vi "Main.vi"(11 "Module Admin":refnum<class "Delacor_lib_QMH_Module Admin.lvclass">) -> ()   [LabVIEW 2025, in "Central Monitor.lvlib"]
doc: "This template is based off of the Queued Message Handler design pattern and the Queued Message Handler project template that ships with LabVIEW.\n\nThe main difference is that the queue is private to this module and communication between modules is performed via Broadcast and Request events.\n\nRequest events are wrapped in public API methods and are handled in the Event Handling Loop (EHL) of this VI. Any module can register for Broadcast events sent by this module. The EHL generates messages based on user interface actions.\n\nThe Message Handling Loop (MHL) processes messages generated by the EHL, or by other messages. The messages are string values, so new messages can be added easily to the Message Cases case structure in the MHL. Each message cluster can also provide an optional value for Message Data, which is a variant that can be converted to whatever message-specific data is required.\n_____\nBased on DQMH Dev Tools: Project Template 7.1.2.1547."
uses:
  Central Monitor.lvlib
  <vilib>/Delacor/Delacor QMH/Libraries/Module Admin_class/Delacor_lib_QMH_Module Admin.lvclass
  Module Data--cluster.ctl
  <vilib>/Delacor/Delacor QMH/Libraries/Message Queue_class/Delacor_lib_QMH_Message Queue.lvclass/Delacor_lib_QMH_Message Queue.ctl
  Stop Argument--cluster.ctl
  <vilib>/Delacor/Delacor QMH/Libraries/Module Admin_class/Delacor_lib_QMH_Module Admin.lvclass/Delacor_lib_QMH_Module Admin.ctl
  <vilib>/Utility/miscctls.llb/LVPointTypeDef.ctl
  <vilib>/Delacor/Delacor QMH/Libraries/Message Queue_class/Delacor_lib_QMH_Enqueue Message (Single).vi
  <vilib>/Delacor/Delacor QMH/Libraries/Module Admin_class/Delacor_lib_QMH_Get External Launch.vi
  <vilib>/Delacor/Delacor QMH/Libraries/Message Queue_class/Delacor_lib_QMH_Message Queue.lvclass
panel:
  in  "Multicolumn Listbox":i32(listbox)
  in  "Button":bool
  out "Monitor Status":bool
  out "Headline":string
  out "error out":errorcluster
  out "Status":string
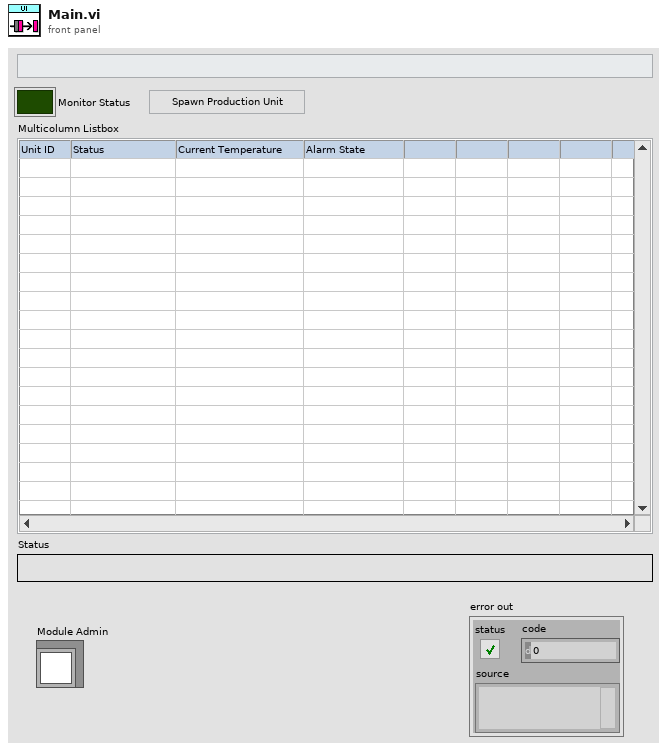
[diagram p1: front panel]
types:
  T1 = typedef "Central Monitor.lvlib/Request Events--cluster.ctl" = cluster{"Stop Module":refnum<user-event>, "Show Panel":refnum<user-event>, "Hide Panel":refnum<user-event>, "Get Module Execution Status":refnum<user-event>, "Show Diagram":refnum<user-event>}
  T2 = typedef "Central Monitor.lvlib/Module Data--cluster.ctl" = cluster{"Status":string}
  T3 = enum32{"invalid lock state", "Not Locked", "Locked (No Password)", "Password-protected"}
  T4 = typedef "Central Monitor.lvlib/Stop Argument--cluster.ctl" = cluster{"Origin":string, "Exit via Stop Module Req?":bool, "Wait for Module to stop?":bool}
  T5 = typedef "LVPointTypeDef.ctl" = cluster{"Horizontal":i16, "Vertical":i16}
  T6 = enum32{"Invalid", "Standard", "Closed", "Hidden", "Minimized", "Maximized"}
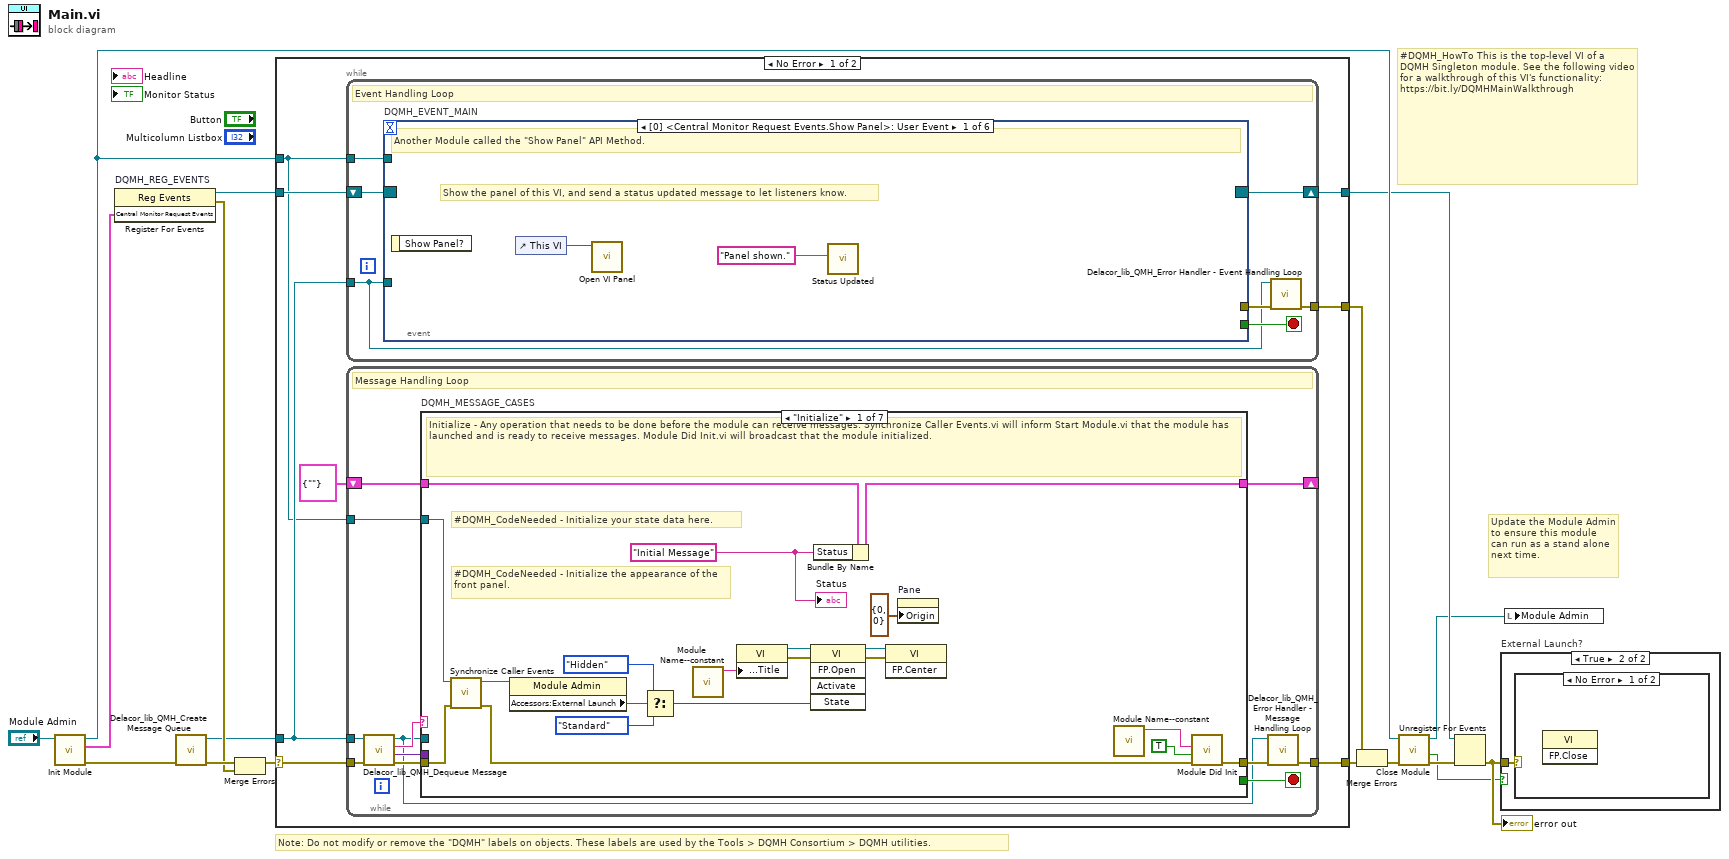
[diagram p0: block diagram]
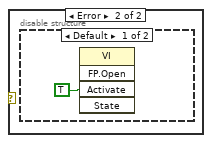
[diagram p3: hidden frame]
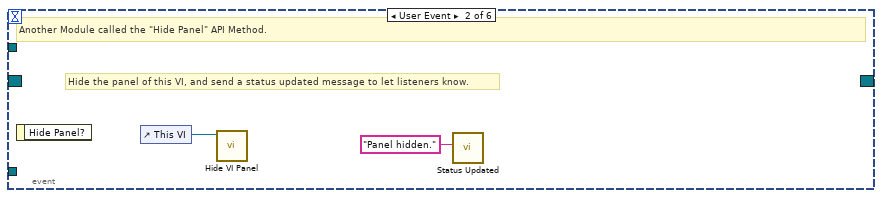
[diagram p5: hidden frame]
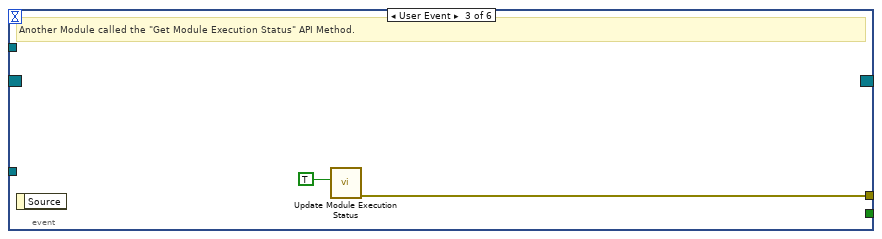
[diagram p6: hidden frame]
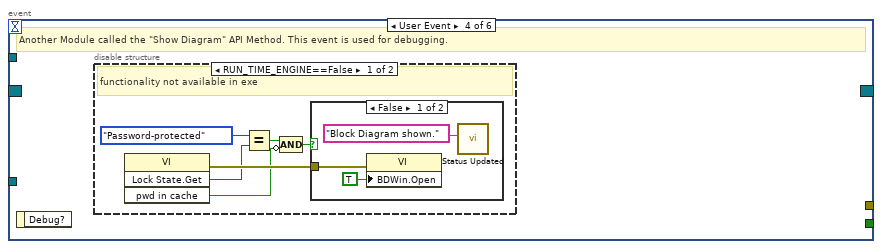
[diagram p7: hidden frame]
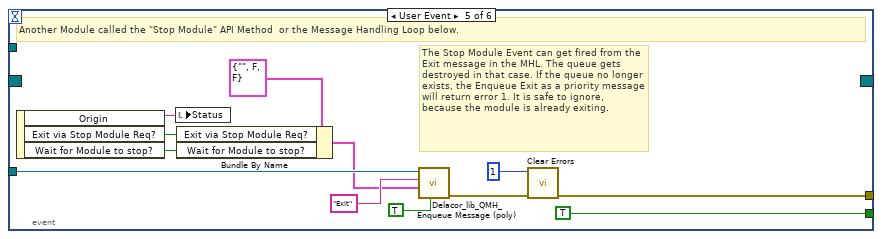
[diagram p10: hidden frame]
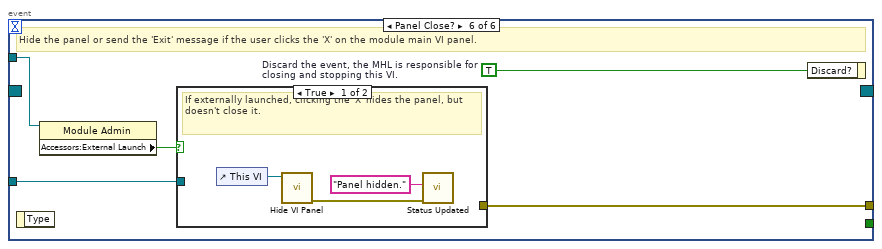
[diagram p11: hidden frame]
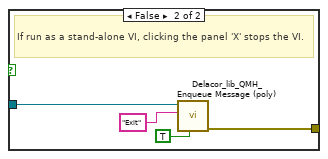
[diagram p12: hidden frame]
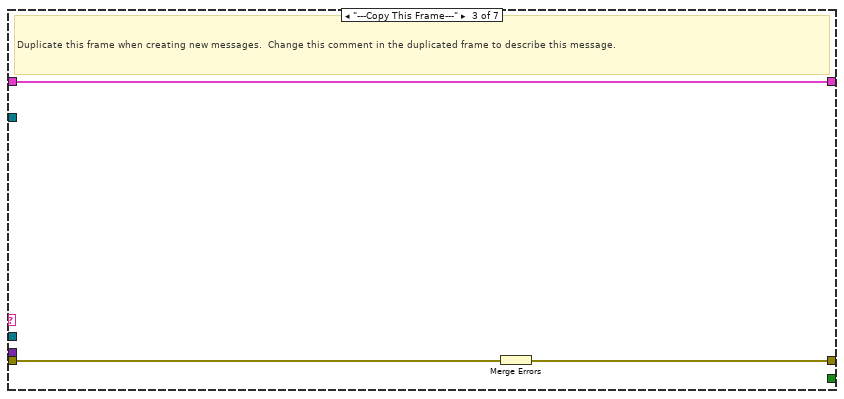
[diagram p14: hidden frame]
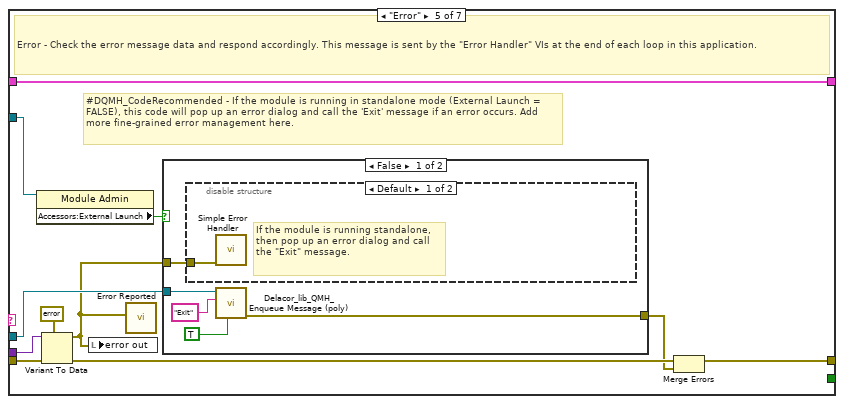
[diagram p16: hidden frame]
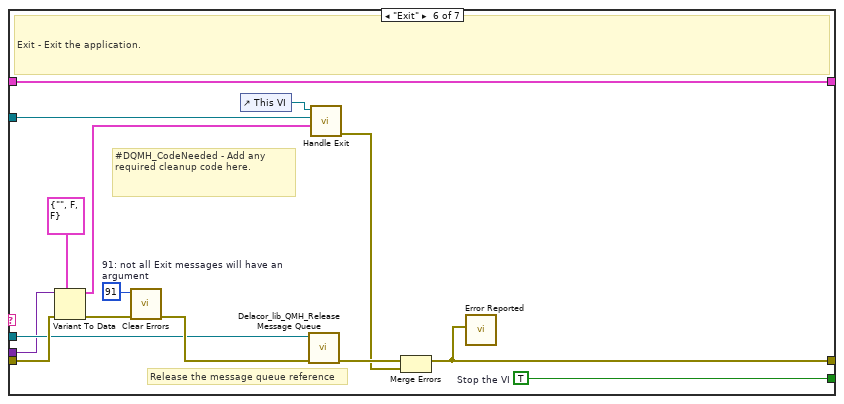
[diagram p19: hidden frame]
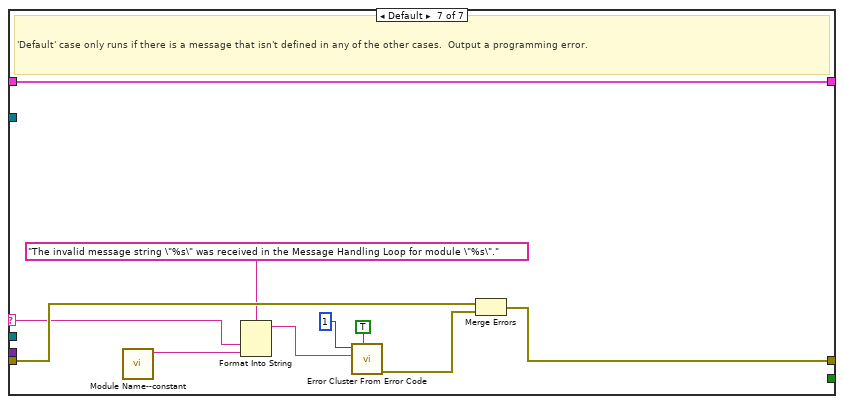
[diagram p20: hidden frame]
diagram:
  # "#DQMH_HowTo This is the top-level VI of a DQMH Singleton module. See the following video for a walkthrough of this VI's functionality: https://bit.ly/DQMHMainWalkthrough"
  # "Note: Do not modify or remove the \"DQMH\" labels on objects. These labels are used by the Tools > DQMH Consortium > DQMH utilities."
  # "Update the Module Admin to ensure this module can run as a stand alone next time."
  n1 = call "Init Module.vi"("Singleton Module Admin in"="Module Admin") -> ("error out"=w16:errorcluster, "Central Monitor Request Events"=w5:T1, "Singleton Module Admin out"=w8:refnum<class "Delacor_lib_QMH_Module Admin.lvclass">)  [unwired: 8 in]
  n2 = register-events "DQMH_REG_EVENTS"(w5) -> (reference out=w6:refnum<event-registration>, error out=w9:errorcluster)  [unwired: 2 in]
  n3 = call <vilib>:"Delacor_lib_QMH_Create Message Queue.vi"("error in"=w16) -> ("error out"=w11:errorcluster, "Message Queue"=w4:refnum<class "Delacor_lib_QMH_Message Queue.lvclass">)  [unwired: 9 in]
  n4 = Merge Errors(w11, w9) -> (w10:errorcluster)
  n5 = case shown="No Error" w10 {
    selector: w10 -> [w23 w160]
    tunnel: [w25 w159] -> w17
    tunnel: [w22 w158] -> w7
    tunnel: w6 -> [w20 w158]
    tunnel: w4 -> [w19 w153]
    tunnel: [w24 _] -> w14
    tunnel: w8 -> [w18 w154]
    frame No Error {
      n6 = while {
        tunnel: w19 -> [w26]
        shift-right: [w29] -> w22
        shift-left: w20 -> [w30]
        tunnel: [w31] -> w24
        tunnel: w18 -> [w27]
        stop <- w28 stop-if-true
        # "Event Handling Loop"
        n7 = event "DQMH_EVENT_MAIN" shown="[0] <Central Monitor Request Events.Show Panel>: User Event" {
          selector: w30 -> [_ _ _ _ _ _]
          dyn-events: [_ _ _ _ _ _] -> w29
          timeout: _ -> [_ _ _ _ _ _]
          tunnel: [_ _ _ _ TRUE ("Discard?") _] -> w28
          tunnel: w26 -> [_ _ _ _ w55 w62]
          tunnel: [_ _ w38 _ w58 w64] -> w32
          tunnel: w27 -> [_ _ _ _ _ w61]
          event User Event {
            # "Show the panel of this VI, and send a status updated message to let listeners know."
            # "Another Module called the \"Show Panel\" API Method."
            n8 = event-data() -> ()  [unwired: 1 in, 1 out]
            n9 = control-ref of="This VI"() -> (w34:refnum<vi>)
            n10 = call "Open VI Panel.vi"("VI"=w34) -> ()  [unwired: 10 in, 1 out]
            n11 = call "Status Updated.vi"("Status"="Panel shown." ("format string")) -> ()  [unwired: 10 in, 1 out]
          }
          event User Event {
            # "Hide the panel of this VI, and send a status updated message to let listeners know."
            # "Another Module called the \"Hide Panel\" API Method."
            n12 = event-data() -> ()  [unwired: 1 in, 1 out]
            n13 = control-ref of="This VI"() -> (w36:refnum<vi>)
            n14 = call "Hide VI Panel.vi"("VI"=w36) -> ()  [unwired: 10 in, 1 out]
            n15 = call "Status Updated.vi"("Status"="Panel hidden." ("format string")) -> ()  [unwired: 10 in, 1 out]
          }
          event User Event {
            # "Another Module called the \"Get Module Execution Status\" API Method."
            n16 = event-data() -> ()  [unwired: 1 in, 1 out]
            n17 = call "Update Module Execution Status.vi"("Running?"=TRUE) -> ("error out"=w38:errorcluster)  [unwired: 10 in]
          }
          event User Event {
            # "Another Module called the \"Show Diagram\" API Method. This event is used for debugging."
            n18 = event-data() -> ()  [unwired: 1 in, 1 out]
            n19 = disable-structure shown="RUN_TIME_ENGINE==False" {
              frame condition #0 (active) {
                # "functionality not available in exe"
                n20 = invoke on="Invoke Node" class="VI" method="Lock State.Get"() -> (error out=w44:errorcluster, "Get Lock State"=w43:T3, "pwd in cache"=w40:bool)  [unwired: 4 in, 1 out]
                n21 = Equal?(x=T3."Password-protected", y=w43) -> (x = y?=w41:bool)
                n22 = Compound Arithmetic op=AND(w41, invert w40) -> (w39:bool)
                n23 = case shown="False" w39 {
                  tunnel: w44 -> [w47 _]
                  frame False {
                    n24 = property on="Property Node" class="VI"(error in=w47, "BDWin.Open"=TRUE ("Block Diagram Window:Open")) -> ()  [unwired: 1 in, 2 out]
                    n25 = call "Status Updated.vi"("Status"="Block Diagram shown." ("format string")) -> ()  [unwired: 10 in, 1 out]
                  }
                  frame True {
                    # "Password-protected VI, and the password is not in the cache. Do not show the diagram."
                  }
                }
              }
              frame condition #1 {
              }
            }
          }
          event User Event {
            # "The Stop Module Event can get fired from the Exit message in the MHL. The queue gets destroyed in that case. If the queue no longer exists, the Enqueue Exit as a priority message will return error 1. It is safe to ignore, because the module is already exiting."
            # "Another Module called the \"Stop Module\" API Method  or the Message Handling Loop below."
            n26 = event-data() -> ("Origin"=w54:string, "Exit via Stop Module Req?"=w50:bool, "Wait for Module to stop?"=w49:bool)  [unwired: 1 in]
            n27 = local write "Status"(w54) -> ()
            n28 = Bundle By Name(cluster=T4 {"Origin"="", "Exit via Stop Module Req?"=FALSE, "Wait for Module to stop?"=FALSE} ("Stop Argument"), "Exit via Stop Module Req?"=w50, "Wait for Module to stop?"=w49) -> (w48:T4)
            n29 = call-poly <vilib>:"Delacor_lib_QMH_Enqueue Message (poly).vi"("Priority Message? (F)"=TRUE, "Message Data"=w48, "Message"="Exit", "Message Queue in"=w55) -> ("error out"=w59:errorcluster)  [unwired: 6 in, 1 out]
            n30 = call <vilib>:"Clear Errors.vi"("error in (no error)"=w59, "specific error code to clear (0: all)"=1) -> ("error out"=w58:errorcluster)  [unwired: 4 in, 1 out]
          }
          event Panel Close? {
            w63 = TRUE  # Discard the event, the MHL is responsible for closing and stopping this VI.
            # "Hide the panel or send the 'Exit' message if the user clicks the 'X' on the module main VI panel."
            n31 = event-data() -> ()  [unwired: 1 in, 1 out]
            n32 = property on="Property Node" class="Module Admin"(reference=w61) -> ("Accessors:External Launch"=w60:bool)  [unwired: 1 in, 2 out]
            n33 = case shown="True" w60 {
              tunnel: w62 -> [_ w70]
              tunnel: [_ w71] -> w64
              frame True {
                # "If externally launched, clicking the 'X' hides the panel, but doesn't close it."
                n34 = control-ref of="This VI"() -> (w67:refnum<vi>)
                n35 = call "Hide VI Panel.vi"("VI"=w67) -> ("error out"=w65:errorcluster)  [unwired: 10 in]
                n36 = call "Status Updated.vi"("error in"=w65, "Status"="Panel hidden." ("format string")) -> ()  [unwired: 9 in, 1 out]
              }
              frame False {
                # "If run as a stand-alone VI, clicking the panel 'X' stops the VI."
                n37 = call-poly <vilib>:"Delacor_lib_QMH_Enqueue Message (poly).vi"("Priority Message? (F)"=TRUE, "Message"="Exit", "Message Queue in"=w70) -> ("error out"=w71:errorcluster)  [unwired: 7 in, 1 out]
              }
            }
            n38 = event-data ("Event Filter Node")("Discard?"=w63) -> ()  [unwired: 1 in, 1 out]
          }
        }
        n39 = call-dynamic "Delacor_lib_QMH_Error Handler - Event Handling Loop.vi"("error in"=w32, "Message Queue in"=w26) -> ("dup error in"=w31:errorcluster)  [unwired: 8 in, 1 out]
      }
      n40 = while {
        tunnel: w19 -> [w72]
        shift-right: [w80] -> _
        shift-left: T2 {"Status"=""} ("Data Cluster") -> [w81]
        tunnel: w23 -> [w83]
        tunnel: [w75] -> w25
        tunnel: w18 -> [w76]
        stop <- w79 stop-if-true
        # "Message Handling Loop"
        n41 = call-dynamic "Delacor_lib_QMH_Dequeue Message.vi"("error in"=w83, "Message Queue in"=w72) -> ("error out"=w82:errorcluster, "Message Data"=w77:variant, "Message"=w78:string, "Message Queue out"=w73:refnum<class "Delacor_lib_QMH_Message Queue.lvclass">)  [unwired: 6 in]
        n42 = case "DQMH_MESSAGE_CASES" shown="\"Initialize\"" w78 {
          selector: w78 -> [_ _ _ _ _ _ w148]
          tunnel: w73 -> [_ _ _ _ w114 w136 _]
          tunnel: w82 -> [w101 w105 w108 w110 w121 w142 w151]
          tunnel: [w99 w105 w107 w110 w117 w137 w152] -> w74
          tunnel: w81 -> [w90 w104 w106 w109 w116 w135 w149]
          tunnel: [w89 w104 w106 w109 w116 w135 w149] -> w80
          tunnel: [_ _ _ _ _ w134 _] -> w79
          tunnel: w77 -> [_ _ _ _ w115 w133 _]
          tunnel: w76 -> [w91 _ _ _ w113 w128 _]
          frame "Initialize" {
            w85 = "Initial Message" ("Initial Message")
            # "#DQMH_CodeNeeded - Initialize the appearance of the front panel."
            # "#DQMH_CodeNeeded - Initialize your state data here."
            # "Initialize - Any operation that needs to be done before the module can receive messages. Synchronize Caller Events.vi will inform Start Module.vi that the module has launched and is ready to receive messages. Module Did Init.vi will broadcast that the module initialized."
            n43 = call "Synchronize Caller Events.vi"("error in"=w101, "Singleton Module Admin in"=w91) -> ("error out"=w100:errorcluster, "Singleton Module Admin out"=w86:refnum<class "Delacor_lib_QMH_Module Admin.lvclass">)  [unwired: 8 in]
            n44 = property on="Property Node" class="Module Admin"(reference=w86) -> ("Accessors:External Launch"=w95:bool)  [unwired: 1 in, 2 out]
            n45 = Select(t=T6."Hidden" ("State"), s=w95, f=T6."Standard" ("State")) -> (s? t:f=w92:T6)
            n46 = call "Module Name--constant.vi"() -> ("Module Name"=w98:string)  [unwired: 11 in]
            n47 = property on="Property Node" class="VI"("Front Panel.Title"=w98) -> (reference out=w97:refnum<vi>, error out=w103:errorcluster)  [unwired: 2 in]
            n48 = invoke on="Invoke Node" class="VI" method="FP.Open"(reference=w97, error in=w103, "State"=w92) -> (reference out=w96:refnum<vi>, error out=w102:errorcluster)  [unwired: 2 in, 3 out]
            n49 = Bundle By Name(cluster=w90, "Status"=w85) -> (w89:T2)
            n50 = invoke on="Invoke Node" class="VI" method="FP.Center"(reference=w96, error in=w102) -> ()  [unwired: 1 in, 3 out]
            n51 = property on="Pane" class="Pane"("Origin"=T5 {"Horizontal"=0, "Vertical"=0}) -> ()  [unwired: 2 in, 2 out]
            n52 = call "Module Name--constant.vi"() -> ("Module Name"=w87:string)  [unwired: 11 in]
            n53 = call "Module Did Init.vi"("error in"=w100, "Initialized?"=TRUE, "Origin"=w87) -> ("error out"=w99:errorcluster)  [unwired: 8 in]
            "Status" <- w85
          }
          frame "---Module Specific---" {
            # "Separator -- The following cases handle messages specific to this Module."
          }
          frame "---Copy This Frame---" {
            # "Duplicate this frame when creating new messages.  Change this comment in the duplicated frame to describe this message."
            n54 = Merge Errors(w108) -> (w107:errorcluster)
          }
          frame "---Exit and Error Handling---" {
            # "Separator - The following cases handle errors and exit messages."
          }
          frame "Error" {
            # "#DQMH_CodeRecommended - If the module is running in standalone mode (External Launch = FALSE), this code will pop up an error dialog and call the 'Exit' message if an error occurs. Add more fine-grained error management here."
            # "Error - Check the error message data and respond accordingly. This message is sent by the \"Error Handler\" VIs at the end of each loop in this application."
            n55 = property on="Property Node" class="Module Admin"(reference=w113) -> ("Accessors:External Launch"=w112:bool)  [unwired: 1 in, 2 out]
            n56 = Variant To Data(error in=w121, type=errorcluster {"status"=FALSE, "code"=0, "source"=""} ("error constant"), Variant=w115) -> (data=w111:errorcluster, error out=w119:errorcluster)
            n57 = local write "error out"(w111) -> ()
            n58 = call "Error Reported.vi"("Error"=w111) -> ()  [unwired: 10 in, 1 out]
            n59 = case shown="False" w112 {
              tunnel: [w126 _] -> w118
              tunnel: w114 -> [w124 _]
              tunnel: w111 -> [w125 _]
              frame False {
                n60 = disable-structure shown="Default" {
                  disable-tunnel: w125 -> [w127 _]
                  frame condition #0 (active) {
                    # "If the module is running standalone, then pop up an error dialog and call the \"Exit\" message."
                    n61 = call <vilib>:"Simple Error Handler.vi"("error in (no error)"=w127) -> ()  [unwired: 4 in, 5 out]
                  }
                  frame condition #1 {
                    # "To prevent the Simple Error Handler VI from being loaded (e.g. when deploying to a Real-Time target), add the Conditional Disable Symbol \"DQMH_Disable_SEH\" to your project and set it to TRUE."
                  }
                }
                n62 = call-poly <vilib>:"Delacor_lib_QMH_Enqueue Message (poly).vi"("Priority Message? (F)"=TRUE, "Message"="Exit", "Message Queue in"=w124) -> ("error out"=w126:errorcluster)  [unwired: 7 in, 1 out]
              }
              frame True {
                # "If the module was launched externally, calling the Error Reported broadcast VI is the only action performed by the \"Error\" message. The module's caller can then process the error appropriately."
              }
            }
            n63 = Merge Errors(w119, w118) -> (w117:errorcluster)
          }
          frame "Exit" {
            w132 = 91  # 91: not all Exit messages will have an argument
            w134 = TRUE  # Stop the VI
            # "Release the message queue reference"
            # "#DQMH_CodeNeeded - Add any required cleanup code here."
            # "Exit - Exit the application."
            n64 = Variant To Data(error in=w142, type=T4 {"Origin"="", "Exit via Stop Module Req?"=FALSE, "Wait for Module to stop?"=FALSE} ("Stop Argument"), Variant=w133) -> (data=w130:T4, error out=w139:errorcluster)
            n65 = call <vilib>:"Clear Errors.vi"("error in (no error)"=w139, "specific error code to clear (0: all)"=w132) -> ("error out"=w141:errorcluster)  [unwired: 4 in, 1 out]
            n66 = control-ref of="This VI"() -> (w129:refnum<vi>)
            n67 = call-dynamic "Delacor_lib_QMH_Release Message Queue.vi"("error in"=w141, "Message Queue"=w136) -> ("error out"=w140:errorcluster)  [unwired: 9 in]
            n68 = call "Handle Exit.vi"("Stop Argument"=w130, "Admin in"=w128, "VI reference"=w129) -> ("error out"=w138:errorcluster)  [unwired: 7 in, 1 out]
            n69 = Merge Errors(w140, w138) -> (w137:errorcluster)
            n70 = call "Error Reported.vi"("Error"=w137) -> ()  [unwired: 10 in, 1 out]
          }
          frame Default {
            # "'Default' case only runs if there is a message that isn't defined in any of the other cases.  Output a programming error."
            n71 = call "Module Name--constant.vi"() -> ("Module Name"=w147:string)  [unwired: 11 in]
            n72 = Format Into String(format string="The invalid message string \"%s\" was received in the Message Handling Loop for module \"%s\".", w148, w147) -> (resulting string=w143:string)  [unwired: 2 in, 1 out]
            n73 = call <vilib>:"Error Cluster From Error Code.vi"("show call chain? (False)"=TRUE, "error message (\"\")"=w143, "error code (0)"=1) -> ("error out"=w150:errorcluster)  [unwired: 6 in]
            n74 = Merge Errors(w151, w150) -> (w152:errorcluster)
          }
        }
        n75 = call-dynamic "Delacor_lib_QMH_Error Handler - Message Handling Loop.vi"("error in"=w74, "Message Queue in"=w73) -> ("dup error in"=w75:errorcluster)  [unwired: 8 in, 1 out]
      }
    }
    frame Error {
      # "Synchronize Caller Events.vi will inform Start Module.vi that the module has launched and will let the code calling Start Module.vi register for broadcasts and would permit the caller receive the broadcast that an error occurred at launch time."
      n76 = call-dynamic "Delacor_lib_QMH_Release Message Queue.vi"("error in"=w160, "Message Queue"=w153) -> ("error out"=w159:errorcluster)  [unwired: 9 in]
      n77 = call "Synchronize Caller Events.vi"("Singleton Module Admin in"=w154) -> ("error out"=w161:errorcluster)  [unwired: 9 in, 1 out]
      n78 = call "Module Name--constant.vi"() -> ("Module Name"=w157:string)  [unwired: 11 in]
      n79 = Format Into String(format string="An error occurred during initialization. %s is no longer running.", w157) -> (resulting string=w155:string)  [unwired: 2 in, 1 out]
      n80 = Merge Errors(w159, w161) -> (w162:errorcluster)
      n81 = call "Error Reported.vi"("Additional Information"=w155, "Error"=w162) -> ()  [unwired: 9 in, 1 out]
    }
  }
  n82 = Merge Errors(w14, w17) -> (w13:errorcluster)
  n83 = call "Close Module.vi"("error in"=w13, "Module Admin in"=w8) -> ("error out"=w15:errorcluster, "External Launch"=w1:bool, "Module Admin out"=w2:refnum<class "Delacor_lib_QMH_Module Admin.lvclass">)  [unwired: 7 in]
  n84 = Unregister For Events(event registration refnum=w7, error in=w15) -> (error out=w12:errorcluster)
  "error out" <- w12
  n85 = case "External Launch?" shown="True" w1 {
    tunnel: w12 -> [_ w163]
    frame False {
    }
    frame True {
      n86 = case shown="No Error" w163 {
        frame No Error {
          n87 = invoke on="Invoke Node" class="VI" method="FP.Close"() -> ()  [unwired: 3 in, 3 out]
        }
        frame Error {
          n88 = disable-structure shown="Default" {
            frame condition #0 (active) {
              n89 = invoke class="VI" method="FP.Open"("Activate"=TRUE ("Activate?")) -> ()  [unwired: 4 in, 5 out]
            }
            frame condition #1 {
              # "Don't show panel on error if running inside a built EXE."
            }
          }
        }
      }
    }
  }
  n90 = local write "Module Admin"(w2) -> ()
